vi "Create Sheep.vi"() -> (3 "Sheep.lvclass":refnum<class "Sheep.lvclass">)   [LabVIEW 2018, in "Sheep.lvclass"]
uses:
  Sheep.lvclass
  animal/Animal.lvclass
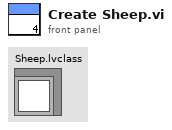
[diagram p1: front panel]
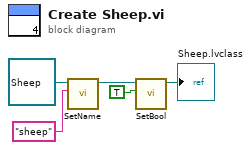
[diagram p0: block diagram]
diagram:
  n1 = call "SetName.vi"("Name"="sheep" ("String"), "Animal in"=refnum<class "Sheep.lvclass"> refnum ("Sheep.lvclass")) -> ("Animal out"=w3:refnum<class "Sheep.lvclass">)  [unwired: 8 in, 1 out]
  n2 = call "SetBool.vi"("Bool"=TRUE, "Animal in"=w3) -> ("Animal out"=→"Sheep.lvclass":refnum<class "Sheep.lvclass">)  [unwired: 8 in, 1 out]
